vi "OxITC503 check temp stability.vi"(0 "Set point proximity":dbl=0.05 format="%.3f", 1 "Stability":dbl=0.05 format="%.3f", 2 "OxfordITC503s":refnum<visa-resource-name>, 3 "seconds to wait":u32=30, 4 "error in":errorcluster) -> (7 "error out":errorcluster)   [LabVIEW 2014]
panel:
  out "Temperature":dbl=26.719 format="%.4f"
  out "Waveform Chart":dbl(graph)=26.719
  out "Set Point":dbl=40.0 format="%.4f"
  in  "Sample time Secs":dbl=1.0
  # "Checking for temperature stability"
  # "Temperature must be within +/-"
  # "of set point"
  # "and stable within +/-"
  # "over"
  # "Seconds"
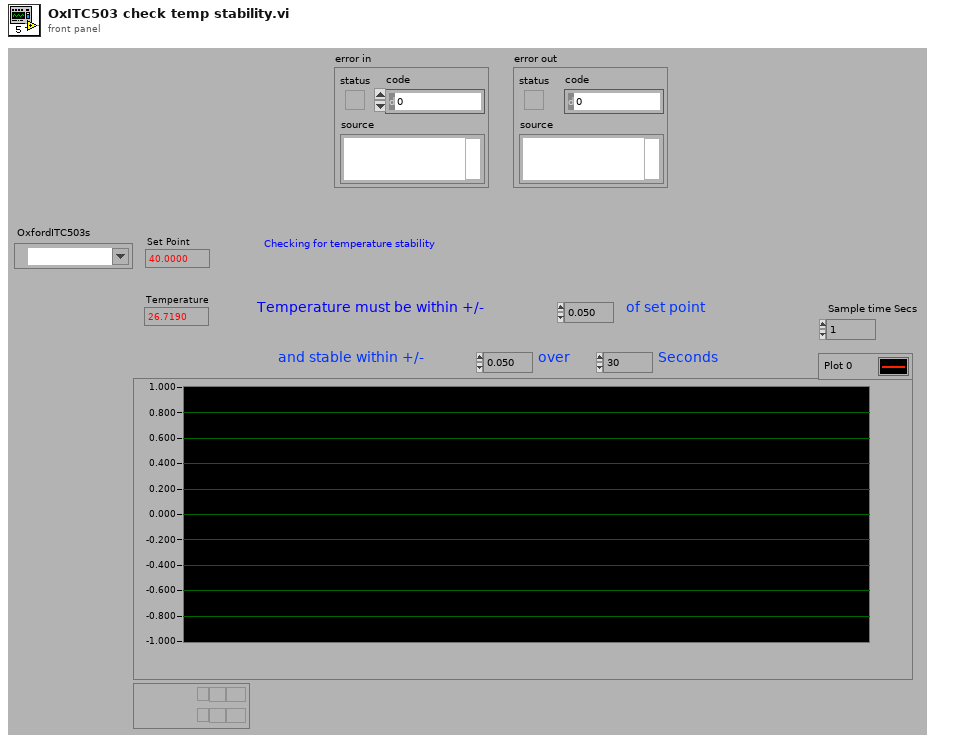
[diagram p1: front panel]
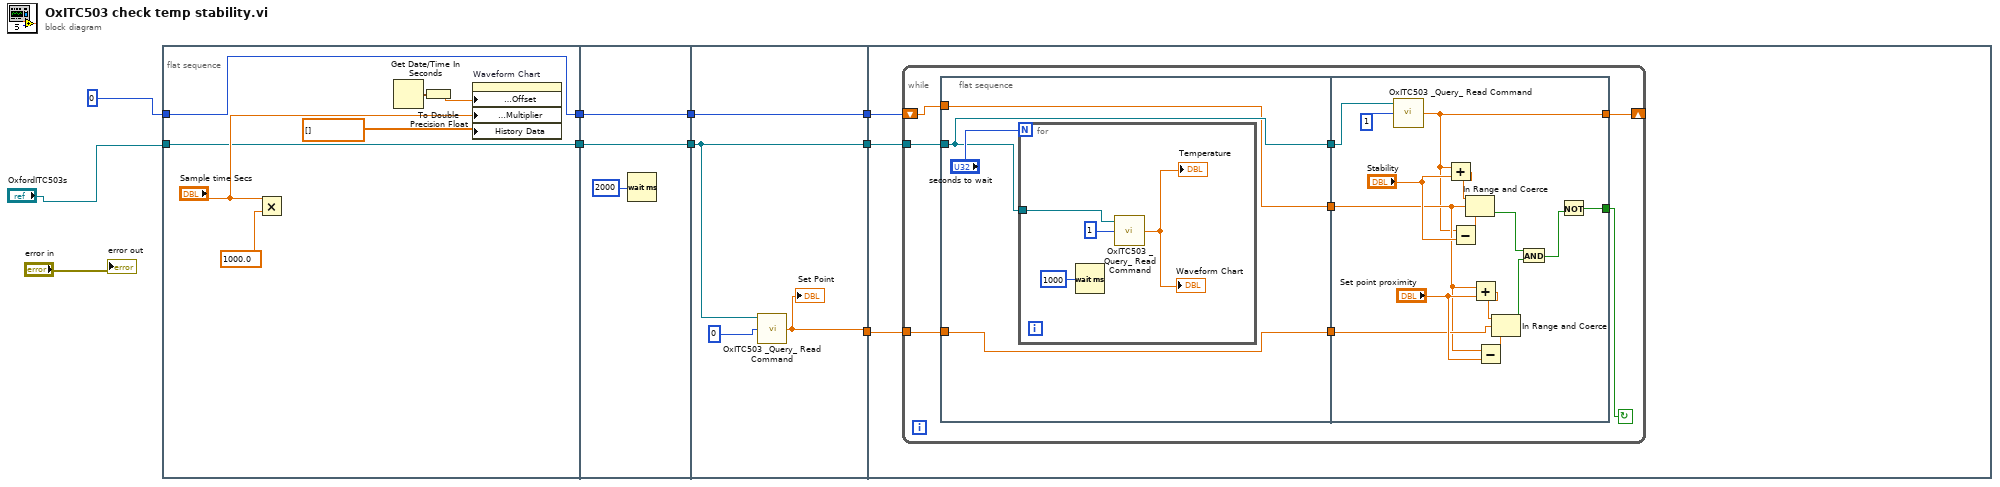
[diagram p0: block diagram]
diagram:
  n1 = flat-sequence {
    tunnel: 0 -> [w12]
    tunnel: [w12] -> w8
    tunnel: "OxfordITC503s" -> [w11]
    tunnel: [w11] -> w7
    tunnel: w8 -> [w19]
    tunnel: [w19] -> w6
    tunnel: w7 -> [w18]
    tunnel: [w18] -> w5
    tunnel: w6 -> [w24]
    tunnel: [w24] -> w4
    tunnel: w5 -> [w23]
    tunnel: [w23] -> w3
    tunnel: [w21] -> w2
    tunnel: w4 -> [w27]
    tunnel: w3 -> [w26]
    tunnel: w2 -> [w25]
    frame #0 {
      n2 = Multiply(x="Sample time Secs", y=1000.0) -> ()  [unwired: 1 out]
      n3 = Get Date/Time In Seconds() -> (seconds since 1Jan1904=w13:timestamp)
      n4 = To Double Precision Float(number=w13) -> (double precision float=w16:dbl)
      n5 = property on="Waveform Chart" class="WFChart (strict)"("X Scale.Offset and Multiplier:Offset"=w16, "X Scale.Offset and Multiplier:Multiplier"="Sample time Secs", "History Data"=dbl[] [] ("Write Attribute")) -> ()  [unwired: 2 in, 2 out]
    }
    frame #1 {
      n6 = Wait (ms)(milliseconds to wait=u32 2000) -> ()  [unwired: 1 out]
    }
    frame #2 {
      n7 = call "OxITC503 _Query_ Read Command.vi"("Read Item"=0, "VISA session"=w23) -> ("Output of Read"=w21:dbl)  [unwired: 1 in, 2 out]
      "Set Point" <- w21
    }
    frame #3 {
      n8 = while {
        tunnel: w25 -> [w31]
        tunnel: w26 -> [w32]
        shift-left: w27 -> [w33]
        shift-right: [w34] -> _
        stop <- w35 continue-if-true
        n9 = flat-sequence {
          tunnel: w33 -> [w37]
          tunnel: [w37] -> w30
          tunnel: w32 -> [w38]
          tunnel: [w38] -> w29
          tunnel: w31 -> [w36]
          tunnel: [w36] -> w28
          tunnel: [w56] -> w35
          tunnel: [w44] -> w34
          tunnel: w30 -> [w47]
          tunnel: w29 -> [w45]
          tunnel: w28 -> [w48]
          frame #0 {
            n10 = for {
              N: "seconds to wait" -> [_]
              tunnel: w38 -> [w42]
              n11 = Wait (ms)(milliseconds to wait=u32 1000) -> ()  [unwired: 1 out]
              n12 = call "OxITC503 _Query_ Read Command.vi"("Read Item"=1, "VISA session"=w42) -> ("Output of Read"=→"Temperature" →"Waveform Chart":dbl)  [unwired: 1 in, 2 out]
            }
          }
          frame #1 {
            n13 = call "OxITC503 _Query_ Read Command.vi"("Read Item"=1, "VISA session"=w45) -> ("Output of Read"=w44:dbl)  [unwired: 1 in, 2 out]
            n14 = Add(x=w44, y="Stability") -> (x+y=w58:dbl)
            n15 = Subtract(x=w44, y="Stability") -> (x-y=w57:dbl)
            n16 = In Range and Coerce(upper limit=w58, x=w47, lower limit=w57) -> (In Range?=w50:bool)  [unwired: 1 out]
            n17 = Add(x=w47, y="Set point proximity") -> (x+y=w54:dbl)
            n18 = Subtract(x=w47, y="Set point proximity") -> (x-y=w53:dbl)
            n19 = In Range and Coerce(upper limit=w54, x=w48, lower limit=w53) -> (In Range?=w52:bool)  [unwired: 1 out]
            n20 = And(x=w50, y=w52) -> (x .and. y?=w49:bool)
            n21 = Not(x=w49) -> (.not. x?=w56:bool)
          }
        }
      }
    }
  }
  "error out" <- "error in"
